vi "NAV_DRIVE_TURN.vi"(7 "arguments":string[](array[string]), 8 "dt":i32, 9 "Reinit":bool, 10 "bus_inputs":T1, 11 "bus_state":T2) -> (1 "Done":bool, 2 "bus_inputs out":T1, 3 "bus_state out":T2)   [LabVIEW 2013]
uses:
  drivetrain/dt_shift_state.ctl
  structures/bus_state_drivetrain.ctl
  structures/bus_state_collector.ctl
  structures/bus_state.ctl
  structures/bus_inputs.ctl
  collector/collector_shot_cal.ctl
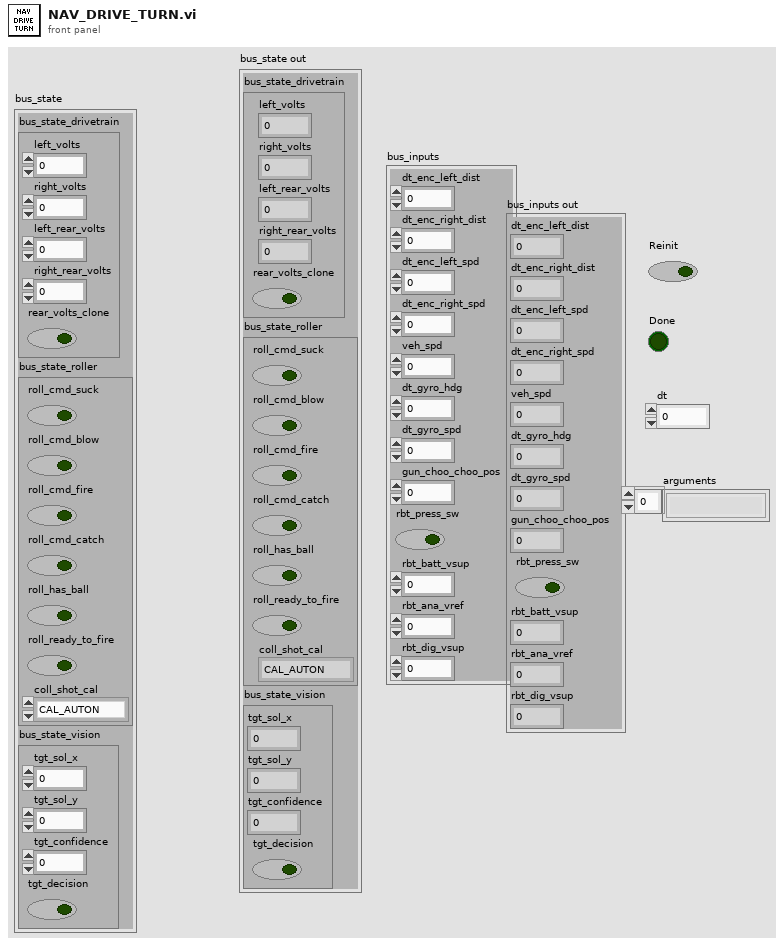
[diagram p1: front panel]
types:
  T1 = typedef "bus_inputs.ctl" = cluster{"dt_enc_left_dist":sgl, "dt_enc_right_dist":sgl, "dt_enc_left_spd":sgl, "dt_enc_right_spd":sgl, "veh_spd":sgl, "dt_gyro_hdg":sgl, "dt_gyro_spd":sgl, "gun_choo_choo_pos":sgl, "rbt_press_sw":bool, "rbt_batt_vsup":sgl, "rbt_ana_vref":dbl, "rbt_dig_vsup":dbl}
  T2 = typedef "bus_state.ctl" = cluster{"bus_state_drivetrain":T3, "bus_state_roller":T4, "bus_state_vision":cluster{"tgt_sol_x":dbl, "tgt_sol_y":dbl, "tgt_confidence":dbl, "tgt_decision":bool}}
  T3 = typedef "bus_state_drivetrain.ctl" = cluster{"left_volts":sgl, "right_volts":sgl, "left_rear_volts":sgl, "right_rear_volts":sgl, "rear_volts_clone":bool}
  T4 = typedef "bus_state_collector.ctl" = cluster{"roll_cmd_suck":bool, "roll_cmd_blow":bool, "roll_cmd_fire":bool, "roll_cmd_catch":bool, "roll_has_ball":bool, "roll_ready_to_fire":bool, "coll_shot_cal":T5}
  T5 = typedef "collector_shot_cal.ctl" = enum16{"CAL_AUTON", "CAL_CLOSE", "CAL_MID", "CAL_FAR"}
  T6 = typedef "dt_shift_state.ctl" = enum16{"low", "high"}
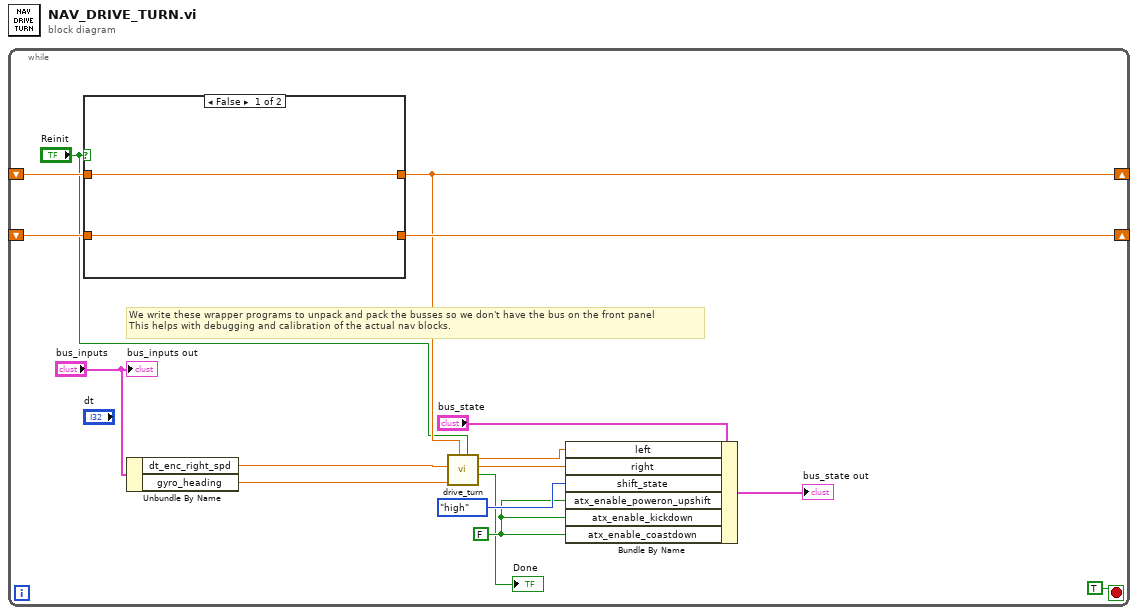
[diagram p0: block diagram]
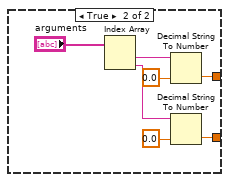
[diagram p2: hidden frame]
diagram:
  n1 = while {
    shift-right: [w2] -> _
    shift-left: _ -> [w15]
    shift-right: [w9] -> _
    shift-left: _ -> [w10]
    stop <- TRUE stop-if-true
    w11 = FALSE ("bus_state_drivetrain.atx_enable_poweron_upshift")
    # "We write these wrapper programs to unpack and pack the busses so we don't have the bus on the front panel\nThis helps with debugging and calibration of the actual nav blocks."
    n2 = case shown="False" "Reinit" {
      tunnel: w15 -> [w18 _]
      tunnel: [w18 w22] -> w2
      tunnel: [w17 w19] -> w9
      tunnel: w10 -> [w17 _]
      frame False {
      }
      frame True {
        n3 = Index Array(array="arguments") -> (element #1=w24:string, element #2=w21:string)  [unwired: 2 in]
        n4 = Decimal String To Number(string=w24, default (0L)=0.0 ("default (0 I32)")) -> (number=w22:dbl)  [unwired: 1 in, 1 out]
        n5 = Decimal String To Number(string=w21, default (0L)=0.0 ("default (0 I32)")) -> (number=w19:dbl)  [unwired: 1 in, 1 out]
      }
    }
    n6 = Unbundle By Name("bus_inputs") -> ("dt_enc_right_spd"=w6:sgl, "gyro_heading"=w5:dbl)
    n7 = call "drive_turn.vi"("reset"="Reinit", "turn_hdg"=w2, "gyro_angle"=w5, "speed_right"=w6) -> ("done"=→"Done":bool, "right"=w3:dbl, "left"=w4:dbl)  [unwired: 5 in]
    n8 = Bundle By Name(cluster="bus_state", "left"=w4, "right"=w3, "shift_state"=dt_shift_state."high" ("bus_state_drivetrain.shift_state"), "atx_enable_poweron_upshift"=w11, "atx_enable_kickdown"=w11, "atx_enable_coastdown"=w11) -> (→"bus_state out":T2)
    "bus_inputs out" <- "bus_inputs"
  }
